vi "IScanOpen.vi"(0 "Port":i32) -> (1 "PRIORLib.IScanOut":refnum<k7>, 2 "error out":errorcluster, 3 "Return":i32)   [LabVIEW 2011]
panel:
  in  "PRIORLib.IScan":refnum<k7>
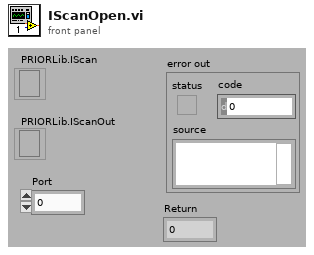
[diagram p1: front panel]
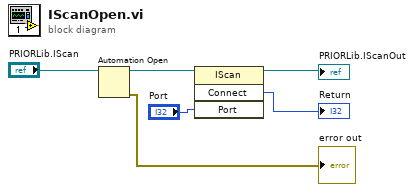
[diagram p0: block diagram]
diagram:
  n1 = Automation Open(Automation Refnum="PRIORLib.IScan") -> (Automation Refnum=w5:refnum<k7>, error out=→"error out":errorcluster)  [unwired: 3 in]
  n2 = invoke class="IScan" method="Connect"(reference=w5, "Port"="Port") -> (reference out=→"PRIORLib.IScanOut":refnum<k7>, "Connect"=→"Return":i32)  [unwired: 2 in, 2 out]
